vi "Read Power.vi"(11 "MCCW ACLR in":refnum<class "MCCW ACLR.lvclass">) -> (2 "Power":cluster{"List":dbl[], "Index":i32, "Last":bool}, 3 "MCCW ACLR out":refnum<class "MCCW ACLR.lvclass">)   [LabVIEW 2020, in "MCCW ACLR.lvclass"]
uses:
  MCCW ACLR.lvclass
  MCCW ACLR.lvclass/MCCW ACLR.ctl
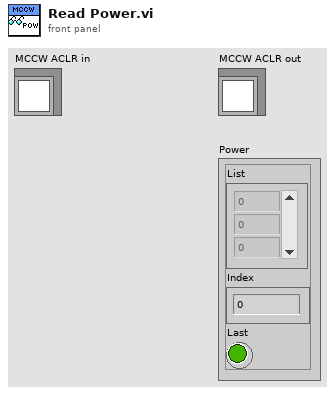
[diagram p1: front panel]
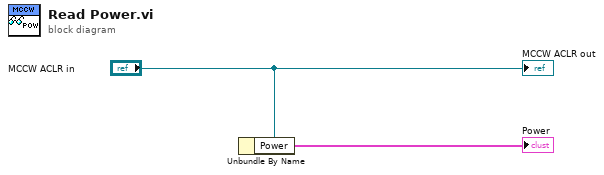
[diagram p0: block diagram]
diagram:
  n1 = Unbundle By Name("MCCW ACLR in") -> ("Power"=→"Power":cluster{"List":dbl[], "Index":i32, "Last":bool})
  "MCCW ACLR out" <- "MCCW ACLR in"
